vi "svfa_Compute Complex Spectrum for Export.vi"(0 "complex spectrum in":T9={"complex spectrum response"={"f0"=0.0, "df"=1.0, "complex spectrum"=[]}, "spectrum info"={"channel name"="", "description"="", "x-axis units"=0, "spectral info"={"spectrum type"=enum."Power [Magnitude^2]", "linear/dB"=enum."linear", "window"=0, "window size"=0, "FFT size"=0}, "engineering units"=0, "custom label"="", "dB reference [EU]"=0.0, "peak units"=enum."rms", "weighting filter"=0, "spectral density?"=FALSE, "unit label"="", "spectrum skewed?"=FALSE, "complimentary spectrum units"=enum."none"}} {"spectrum info"."x-axis units" items=["Time (s)"=0, "Frequency-CB (Hz)"=1, "Frequency-CPB (Hz)"=1248, "Frequency-Arbitrary (Hz)"=2357, "Quefrency (s)"=2, "Revolutions (rev)"=3, "Order"=4, "Speed (RPM)"=11, "Speed (rad/s)"=21, "Index"=65535]; "spectrum info"."weighting filter" items=["Linear", "A-weighting", "B-weighting", "C-weighting", "ITU-R 468-4", "Dolby", "CCITT", "C-message", "Wb", "Wc", "Wd", "We", "Wf", "Wh", "Wj", "Wk", "Wm", "AES17 20 kHz lowpass", "AES17 40 kHz lowpass", "AES17 20 kHz highpass", "AES17 40 kHz highpass"]; "spectrum info"."dB reference [EU]" format="%.2f"; "spectrum info"."engineering units" items=["custom..."=0, "V"=1, "A"=21, "C"=30, "pC"=31, "s"=32, "-"=29, "Pa"=2, "N"=20, "g"=3, "m/s^2"=4, "m/s"=5, "m"=6, "mm/s"=12, "mm"=13, "micron/s"=14, "micron"=15, "in/s^2"=7, "in/s"=8, "in"=9, "mil/s"=10, "mil"=11, "rad/s^2"=16, "rad/s"=17, "rad"=18, "deg/s^2"=26, "deg/s"=27, "deg"=28, "RPM"=22, "cycle/s^2"=23, "Hz"=24, "cycle"=25, "strain"=19]; "spectrum info"."spectral info"."window" items=["None "=0, "Hanning"=1, "Hamming"=2, "Blackman-Harris"=3, "Exact Blackman"=4, "Blackman"=5, "Flat Top"=6, "4 Term B-Harris "=7, "7 Term B-Harris"=8, "Low Sidelobe"=9, "Force - Exponential"=10, "Gaussian"=62]; "complex spectrum response"."complex spectrum" format="%.2f"; "complex spectrum response"."df" format="%.2f"; "complex spectrum response"."f0" format="%.2f"}, 1 "tones":T1(array[cluster]) {"phase (deg)" format="%0.3p"; "amplitude [EU pk]" format="%0.3p"; "frequency [Hz]" format="%0.3p"}, 3 "advanced span [Hz]":dbl=-1.0, 5 "error in":errorcluster, 6 "export signals":T2(ring)) -> (14 "complex spectrum out":T9={"complex spectrum response"={"f0"=0.0, "df"=1.0, "complex spectrum"=[]}, "spectrum info"={"channel name"="", "description"="", "x-axis units"=0, "spectral info"={"spectrum type"=enum."Power [Magnitude^2]", "linear/dB"=enum."linear", "window"=0, "window size"=0, "FFT size"=0}, "engineering units"=0, "custom label"="", "dB reference [EU]"=0.0, "peak units"=enum."rms", "weighting filter"=0, "spectral density?"=FALSE, "unit label"="", "spectrum skewed?"=FALSE, "complimentary spectrum units"=enum."none"}} {"spectrum info"."x-axis units" items=["Time (s)"=0, "Frequency-CB (Hz)"=1, "Frequency-CPB (Hz)"=1248, "Frequency-Arbitrary (Hz)"=2357, "Quefrency (s)"=2, "Revolutions (rev)"=3, "Order"=4, "Speed (RPM)"=11, "Speed (rad/s)"=21, "Index"=65535]; "spectrum info"."weighting filter" items=["Linear", "A-weighting", "B-weighting", "C-weighting", "ITU-R 468-4", "Dolby", "CCITT", "C-message", "Wb", "Wc", "Wd", "We", "Wf", "Wh", "Wj", "Wk", "Wm", "AES17 20 kHz lowpass", "AES17 40 kHz lowpass", "AES17 20 kHz highpass", "AES17 40 kHz highpass"]; "spectrum info"."dB reference [EU]" format="%.2f"; "spectrum info"."engineering units" items=["custom..."=0, "V"=1, "A"=21, "C"=30, "pC"=31, "s"=32, "-"=29, "Pa"=2, "N"=20, "g"=3, "m/s^2"=4, "m/s"=5, "m"=6, "mm/s"=12, "mm"=13, "micron/s"=14, "micron"=15, "in/s^2"=7, "in/s"=8, "in"=9, "mil/s"=10, "mil"=11, "rad/s^2"=16, "rad/s"=17, "rad"=18, "deg/s^2"=26, "deg/s"=27, "deg"=28, "RPM"=22, "cycle/s^2"=23, "Hz"=24, "cycle"=25, "strain"=19]; "spectrum info"."spectral info"."window" items=["None "=0, "Hanning"=1, "Hamming"=2, "Blackman-Harris"=3, "Exact Blackman"=4, "Blackman"=5, "Flat Top"=6, "4 Term B-Harris "=7, "7 Term B-Harris"=8, "Low Sidelobe"=9, "Force - Exponential"=10, "Gaussian"=62]; "complex spectrum response"."complex spectrum" format="%.2f"; "complex spectrum response"."df" format="%.2f"; "complex spectrum response"."f0" format="%.2f"}, 17 "residual bandwidth ratio":dbl=1.0 format="%_6g", 19 "error out":errorcluster)   [LabVIEW 2017]
uses:
  <vilib>/addons/_NISVFA/_Shared subVIs/Controls/svc_Spectrum Info.ctl
  <vilib>/addons/_NISVFA/_Shared subVIs/Controls/svc_X-Axis Units.ctl
  <vilib>/addons/_NISVFA/_Shared subVIs/Controls/svc_Spectrum Type.ctl
  <vilib>/addons/_NISVFA/_Shared subVIs/Controls/svc_Engineering Units Text Ring.ctl
  <vilib>/addons/_NISVFA/_Shared subVIs/Controls/svc_Weighting Filter Text Ring.ctl
  <vilib>/addons/_NISVFA/_Shared subVIs/Controls/svc_Complimentary Spectrum Units.ctl
  <vilib>/addons/_NISVFA/_Spectrum Processing/SVFA Get Spectrum Subset (Complex) (1 Ch).vi
  <vilib>/measure/NI_MABase.lvlib
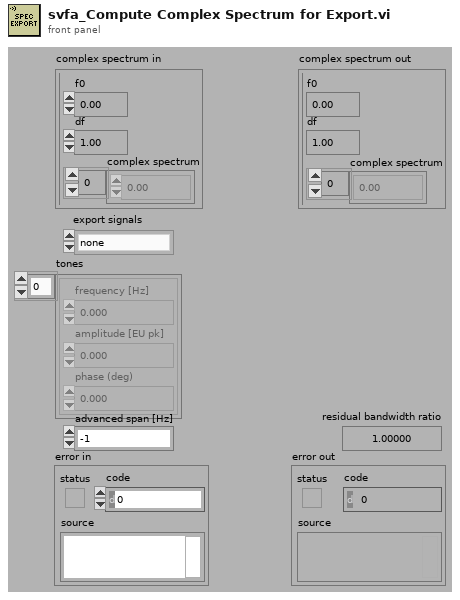
[diagram p1: front panel]
types:
  T1 = cluster{"frequency [Hz]":dbl, "amplitude [EU pk]":dbl, "phase (deg)":dbl}[]
  T2 = enum32{"none", "input signal", "detected signal", "residual signal"}
  T3 = typedef "svc_Spectrum Info.ctl" = cluster{"channel name":string, "description":string, "x-axis units":T4, "spectral info":cluster{"spectrum type":T5, "linear/dB":enum16{"linear", "dB"}, "window":u16, "window size":i32, "FFT size":i32}, "engineering units":T6, "custom label":string, "dB reference [EU]":dbl, "peak units":enum16{"rms", "peak", "peak-peak"}, "weighting filter":T7, "spectral density?":bool, "unit label":string, "spectrum skewed?":bool, "complimentary spectrum units":T8}
  T4 = typedef "svc_X-Axis Units.ctl" = u16
  T5 = typedef "svc_Spectrum Type.ctl" = enum16{"FFT Spectrum [complex]", "Amplitude [Magnitude]", "Power [Magnitude^2]", "Cross Spectrum [complex]", "Frequency Response [Complex]"}
  T6 = typedef "svc_Engineering Units Text Ring.ctl" = u16
  T7 = typedef "svc_Weighting Filter Text Ring.ctl" = u16
  T8 = typedef "svc_Complimentary Spectrum Units.ctl" = enum16{"none", "radians", "degrees", "cycles", "imaginary"}
  T9 = cluster{"complex spectrum response":cluster{"f0":dbl, "df":dbl, "complex spectrum":cdb[]}, "spectrum info":T3}
  T10 = cluster{"complex spectrum subset":cluster{"x0":dbl, "dx":dbl, "complex array":cdb[]}, "spectrum info":T3}
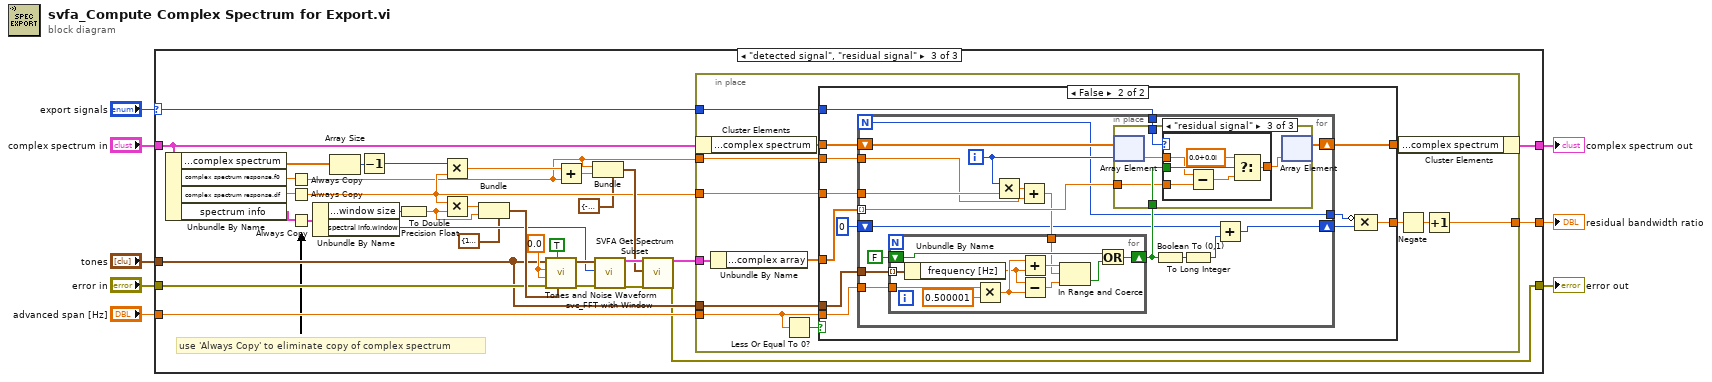
[diagram p0: block diagram]
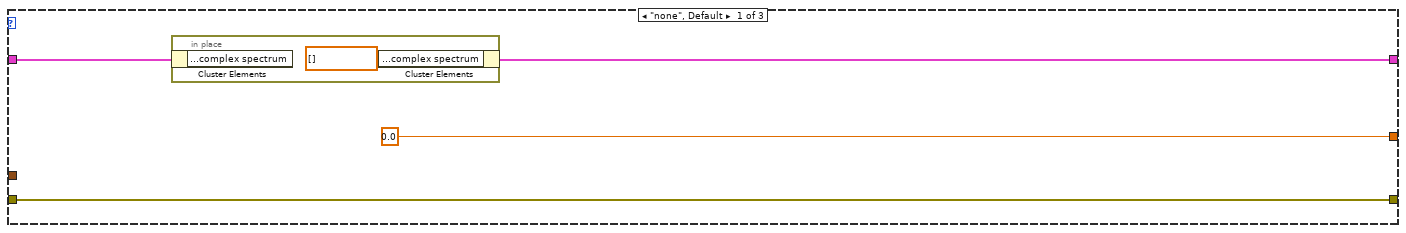
[diagram p2: hidden frame]
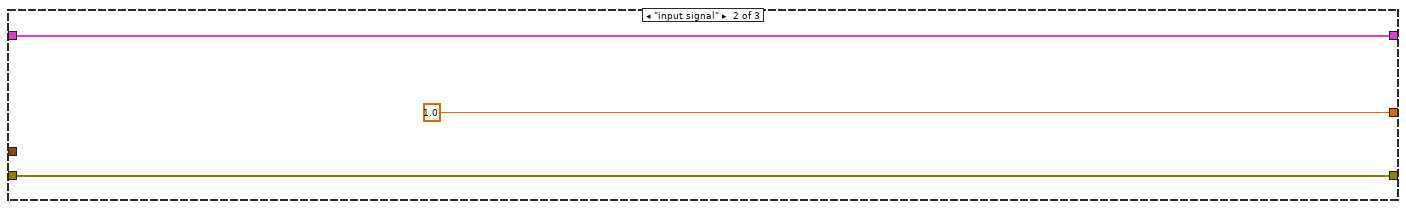
[diagram p3: hidden frame]
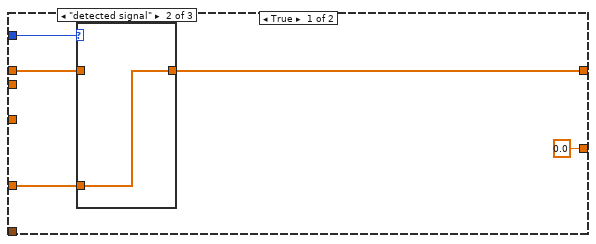
[diagram p4: hidden frame]
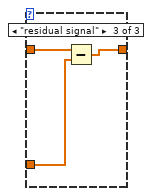
[diagram p6: hidden frame]
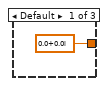
[diagram p7: hidden frame]
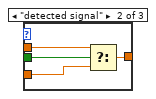
[diagram p8: hidden frame]
diagram:
  n1 = case shown="\"detected signal\", \"residual signal\"" "export signals" {
    selector: "export signals" -> [_ _ w43]
    tunnel: [w11 w16 w24] -> w5
    tunnel: "complex spectrum in" -> [w12 w16 w25]
    tunnel: [w10 w15 w20] -> w6
    tunnel: "error in" -> [w10 w15 w38]
    tunnel: "tones" -> [_ _ w34]
    tunnel: "advanced span [Hz]" -> [_ _ w35]
    tunnel: [0.0 1.0 w17] -> w1
    frame "none", Default {
      n2 = in-place {
        n3 = in-place-cluster #1(w12) -> ()  [unwired: 1 out]
        n4 = in-place-cluster #1("complex spectrum response.complex spectrum"=cdb[] []) -> (w11:T9)
      }
    }
    frame "input signal" {
    }
    frame "detected signal", "residual signal" {
      w41 = 0.0 ("noise (rms)")
      # "use 'Always Copy' to eliminate copy of complex spectrum"
      n5 = Unbundle By Name(w25) -> ("complex spectrum response.complex spectrum"=w30:cdb[], "complex spectrum response.f0"=w29:dbl, "complex spectrum response.df"=w28:dbl, "spectrum info"=w27:T3)
      n6 = Always Copy(1:w29) -> (0:w21:dbl)
      n7 = Always Copy(1:w28) -> (0:w22:dbl)
      n8 = Always Copy(1:w27) -> (0:w23:T3)
      n9 = Unbundle By Name(w23) -> ("spectral info.window size"=w33:i32, "spectral info.window"=w32:u16)
      n10 = Array Size(array=w30) -> (size(s)=w44:i32)
      n11 = Decrement(x=w44) -> (x-1=w50:i32)
      n12 = To Double Precision Float(number=w33) -> (double precision float=w31:dbl)
      n13 = Multiply(x=w50, y=w22) -> (x*y=w49:dbl)
      n14 = Multiply(x=w22, y=w31) -> (x*y=w42:dbl)
      n15 = Bundle(cluster=cluster{"Fs":dbl, "#s":dbl} {"Fs"=1000.0, "#s"=1000.0} ("sampling info"), "Fs"=w42, "#s"=w31) -> (w39:cluster{"Fs":dbl, "#s":dbl})
      n16 = call <vilib>:"Tones and Noise Waveform.vi"("sampling info"=w39, "reset signal"=TRUE, "error in (no error)"=w38, "offset"=w41, "noise (rms)"=w41, "tones"=w34) -> ("error out"=w37:errorcluster, "signal out"=w36:waveform(dbl))  [unwired: 4 in]
      n17 = Add(x=w49, y=w21) -> (x+y=w46:dbl)
      n18 = Bundle(cluster=cluster{"start":dbl, "stop":dbl} {"start"=-1.0, "stop"=-1.0} ("range"), "start"=w21, "stop"=w46) -> (w45:cluster{"start":dbl, "stop":dbl})
      n19 = call <vilib>:"svc_FFT with Window.vi"("time signal in [EU]"=w36, "window"=w32, "error in (no error)"=w37) -> ("complex spectrum"=w47:T9, "error out"=w48:errorcluster)  [unwired: 15 in]
      n20 = call-poly <vilib>:"SVFA Get Spectrum Subset.vi"("complex spectrum"=w47, "range"=w45, "error in (no error)"=w48) -> ("complex spectrum subset"=w26:T10, "error out"=w20:errorcluster)  [unwired: 13 in, 2 out]
      n21 = in-place {
        in-place-border: w43 -> [w63]
        in-place-border: w35 -> [w54]
        in-place-border: w34 -> [w62]
        in-place-border: w21 -> [w61]
        in-place-border: w22 -> [w60]
        in-place-border: w26 -> [w59]
        in-place-border: [w51] -> w17
        n22 = in-place-cluster #2(w25) -> ("complex spectrum response.complex spectrum"=w57:cdb[])
        n23 = Unbundle By Name(w59) -> ("complex spectrum subset.complex array"=w58:cdb[])
        n24 = Less Or Equal To 0?(x=w54) -> (x <= 0?=w55:bool)
        n25 = case shown="False" w55 {
          tunnel: w57 -> [w66 w79]
          tunnel: w63 -> [w68 w83]
          tunnel: w54 -> [_ w84]
          tunnel: w62 -> [_ w85]
          tunnel: w61 -> [_ w81]
          tunnel: w60 -> [_ w82]
          tunnel: w58 -> [w67 w80]
          tunnel: [w65 w78] -> w56
          tunnel: [0.0 w74] -> w53
          frame True {
            n26 = case shown="\"detected signal\"" w68 {
              tunnel: [w69 w70 w71] -> w65
              tunnel: w66 -> [w69 _ w73]
              tunnel: w67 -> [_ w70 w72]
              frame Default {
              }
              frame "detected signal" {
              }
              frame "residual signal" {
                n27 = Subtract(x=w73, y=w72) -> (x-y=w71:cdb[])
              }
            }
          }
          frame False {
            n28 = for {
              N -> [w86]
              tunnel: w85 -> [w103]
              tunnel: w84 -> [w102]
              tunnel: w83 -> [w100]
              tunnel: w80 -> [w99] mode=indexing
              shift-right: [w97] -> w78
              shift-left: w79 -> [w98]
              tunnel: w82 -> [w95]
              tunnel: w81 -> [w92]
              shift-right: [w88] -> w76
              shift-left: 0 -> [w87]
              tunnel: [w86] -> w75
              i -> [w96]
              n29 = Multiply(x=w96, y=w95) -> (x*y=w94:dbl)
              n30 = Add(x=w94, y=w92) -> (x+y=w93:dbl)
              n31 = for {
                tunnel: w103 -> [w130] mode=indexing
                tunnel: w102 -> [w127]
                shift-right: [w120] -> w91
                shift-left: FALSE ("reset signal") -> [w123]
                tunnel: w93 -> [w122]
                n32 = Unbundle By Name(w130) -> ("frequency [Hz]"=w126:dbl)
                n33 = Multiply(x=w127, y=0.500001 ("value")) -> (x*y=w128:dbl)
                n34 = Add(x=w128, y=w126) -> (x+y=w125:dbl)
                n35 = Subtract(x=w126, y=w128) -> (x-y=w124:dbl)
                n36 = In Range and Coerce(upper limit=w125, x=w122, lower limit=w124) -> (In Range?=w121:bool)  [unwired: 1 out]
                n37 = Or(x=w123, y=w121) -> (x .or. y?=w120:bool)
              }
              n38 = in-place {
                in-place-border: w91 -> [w108]
                in-place-border: w100 -> [w107]
                in-place-border: w99 -> [w106]
                n39 = in-place-array #3(w98, w96) -> (w105:cdb)
                n40 = case shown="\"residual signal\"" w107 {
                  tunnel: w108 -> [_ w112 w119]
                  tunnel: [cdb 0.0+0.0i ("t") w113 w118] -> w104
                  tunnel: w105 -> [_ w111 w116]
                  tunnel: w106 -> [_ w110 w115]
                  frame Default {
                  }
                  frame "detected signal" {
                    n41 = Select(t=w111, s=w112, f=w110) -> (s? t:f=w113:cdb)
                  }
                  frame "residual signal" {
                    n42 = Subtract(x=w116, y=w115) -> (x-y=w117:cdb)
                    n43 = Select(t=cdb 0.0+0.0i, s=w119, f=w117) -> (s? t:f=w118:cdb)
                  }
                }
                n44 = in-place-array #3(w104) -> (w97:cdb[])  [unwired: 1 out]
              }
              n45 = Boolean To (0,1)(Boolean=w91) -> (0, 1=w90:i16)
              n46 = To Long Integer(number=w90) -> (32bit integer=w89:i32)
              n47 = Add(x=w87, y=w89) -> (x+y=w88:i32)
            }
            n48 = Compound Arithmetic op=MULTIPLY(invert w75, w76) -> (w74:dbl)
          }
        }
        n49 = Negate(x=w53) -> (-x=w52:dbl)
        n50 = in-place-cluster #2("complex spectrum response.complex spectrum"=w56) -> (w24:T9)
        n51 = Increment(x=w52) -> (x+1=w51:dbl)
      }
    }
  }
  "error out" <- w6
  "complex spectrum out" <- w5
  "residual bandwidth ratio" <- w1
